vi "FTP_STOR.vi"(5 "file path":path, 6 "error in":errorcluster, 7 "Passive Port":T1, 8 "Remote Path":string, 9 "connection ID":refnum<k5>) -> (0 "error out":errorcluster, 1 "Good Reply?":bool, 2 "reply string":string, 3 "connection ID out":refnum<k5>)   [LabVIEW 2012]
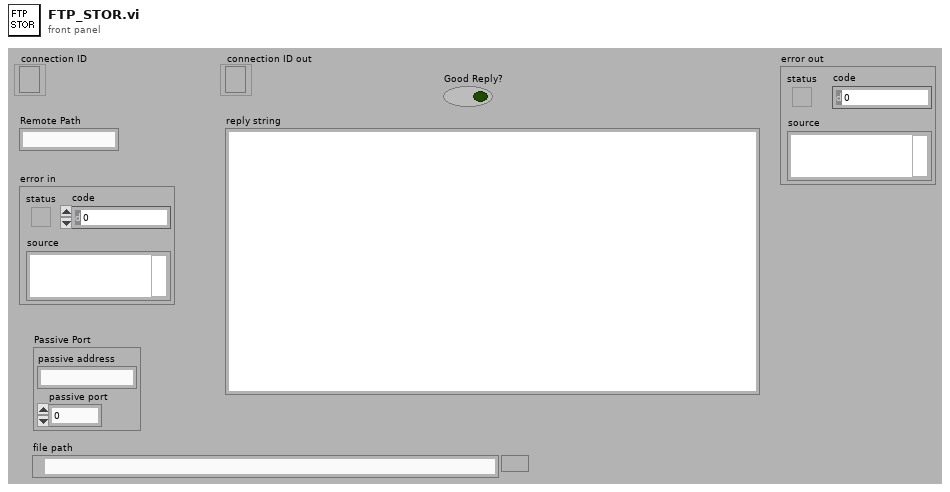
[diagram p1: front panel]
types:
  T1 = cluster{"passive address":string, "passive port":u16}
  T2 = enum16{"unknown", "100 + Prelim", "200 + ", "300 + Intermed", "400 - Transient", "500 - Permanent"}
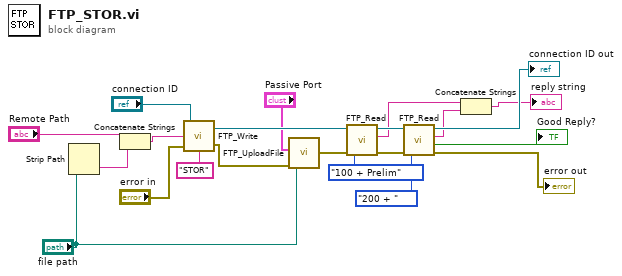
[diagram p0: block diagram]
diagram:
  n1 = Strip Path(path="file path") -> (name=w14:string)  [unwired: 1 out]
  n2 = Concatenate Strings("Remote Path", w14) -> (w12:string)
  n3 = call <userlib>:"FTP_Write.vi"("Cmd"="STOR", "error in"="error in", "data"=w12, "connection ID in"="connection ID") -> ("error out"=w15:errorcluster, "connection ID out"=w18:refnum<k5>)
  n4 = call <userlib>:"FTP_UploadFile.vi"("error in"=w15, "Passive Port"="Passive Port", "file path"="file path") -> ("error out"=w10:errorcluster)  [unwired: 1 in]
  n5 = call <userlib>:"FTP_Read.vi"("error In"=w10, "expected class"=T2."100 + Prelim", "connection ID"=w18) -> ("error out"=w3:errorcluster, "reply string"=w5:string, "connection ID out"=w9:refnum<k5>)  [unwired: 2 out]
  n6 = call <userlib>:"FTP_Read.vi"("error In"=w3, "expected class"=T2."200 + ", "connection ID"=w9) -> ("error out"=→"error out":errorcluster, "Good Reply?"=→"Good Reply?":bool, "reply string"=w6:string, "connection ID out"=→"connection ID out":refnum<k5>)  [unwired: 1 out]
  n7 = Concatenate Strings(w5, w6) -> (→"reply string":string)
